vi "Write Pass_.vi"(8 "error in (no error)":errorcluster, 10 "Pass?":bool, 11 "BallInterception in":refnum<class "BallInterception.lvclass">) -> (0 "error out":errorcluster, 3 "BallInterception out":refnum<class "BallInterception.lvclass">)   [LabVIEW 2023, in "BallInterception.lvclass"]
uses:
  BallInterception.lvclass
  BallInterception.lvclass/BallInterception.ctl
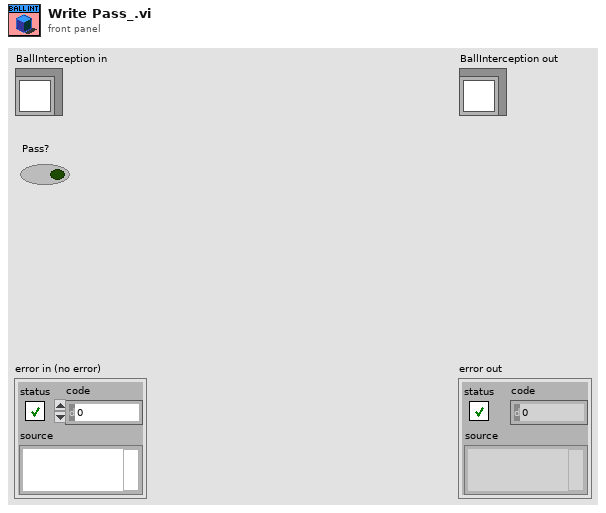
[diagram p1: front panel]
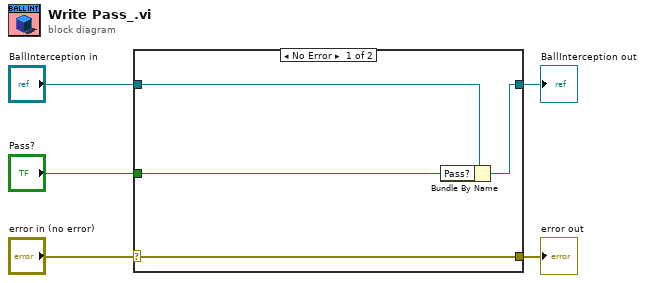
[diagram p0: block diagram]
diagram:
  n1 = case shown="No Error" "error in (no error)" {
    selector: "error in (no error)" -> [w9 w10]
    tunnel: [w9 w10] -> w4
    tunnel: [w7 w11] -> w2
    tunnel: "BallInterception in" -> [w8 w11]
    tunnel: "Pass?" -> [w6 _]
    frame No Error {
      n2 = Bundle By Name(cluster=w8, "Pass?"=w6) -> (w7:refnum<class "BallInterception.lvclass">)
    }
    frame Error {
    }
  }
  "error out" <- w4
  "BallInterception out" <- w2
